vi "writeMisc.vi"(8 "error in (no error)":errorcluster, 9 "Misc":T1, 10 "Pod Number":i32, 11 "Refnum in":T2) -> (0 "error out":errorcluster, 3 "Refnum out":T2)   [LabVIEW 2014]
uses:
  <vilib>/Utility/config.llb/Config Data RefNum.ctl
  <vilib>/Utility/config.llb/Write Key (I32).vi
  <vilib>/Utility/config.llb/Write Key (Double).vi
  <vilib>/Utility/config.llb/NI_LVConfig.lvlib
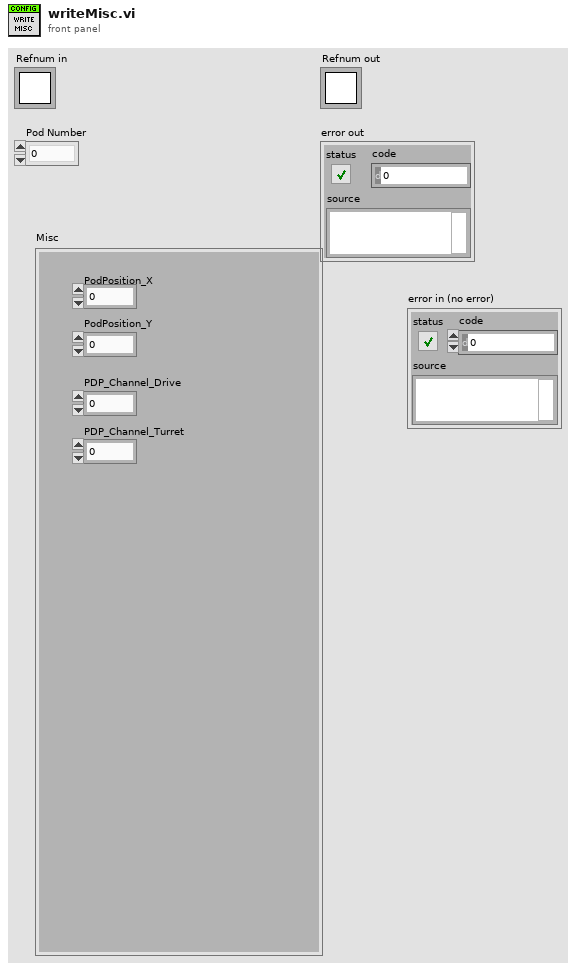
[diagram p1: front panel]
types:
  T1 = cluster{"PodPosition_X":dbl, "PodPosition_Y":dbl, "PDP_Channel_Drive":i32, "PDP_Channel_Turret":i32}
  T2 = typedef "NI_LVConfig.lvlib/Config Data RefNum.ctl" = refnum<k1>
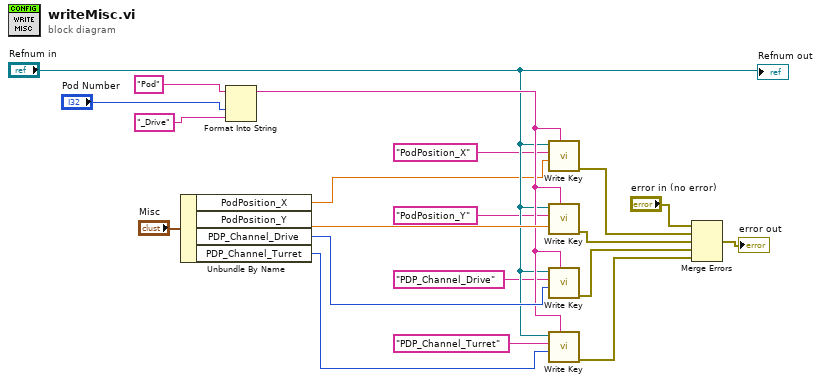
[diagram p0: block diagram]
diagram:
  n1 = Unbundle By Name("Misc") -> ("PodPosition_X"=w4:dbl, "PodPosition_Y"=w16:dbl, "PDP_Channel_Drive"=w14:i32, "PDP_Channel_Turret"=w15:i32)
  n2 = Format Into String(initial string="Pod", "Pod Number", "_Drive") -> (resulting string=w13:string)  [unwired: 2 in, 1 out]
  n3 = call-poly <vilib>:"Write Key.vi"("section"=w13, "value"=w4, "key"="PodPosition_X", "refnum"="Refnum in") -> ("error out"=w17:errorcluster)  [unwired: 5 in, 2 out]
  n4 = call-poly <vilib>:"Write Key.vi"("section"=w13, "value"=w16, "key"="PodPosition_Y", "refnum"="Refnum in") -> ("error out"=w18:errorcluster)  [unwired: 5 in, 2 out]
  n5 = call-poly <vilib>:"Write Key.vi"("section"=w13, "value"=w14, "key"="PDP_Channel_Drive", "refnum"="Refnum in") -> ("error out"=w19:errorcluster)  [unwired: 5 in, 2 out]
  n6 = call-poly <vilib>:"Write Key.vi"("section"=w13, "value"=w15, "key"="PDP_Channel_Turret", "refnum"="Refnum in") -> ("error out"=w2:errorcluster)  [unwired: 5 in, 2 out]
  n7 = Merge Errors("error in (no error)", w17, w18, w19, w2) -> (→"error out":errorcluster)
  "Refnum out" <- "Refnum in"
